vi "gds_rx_init.vi"(8 "error in (no error)":errorcluster, 10 "HW parameters In":T2={"Device IP Address"="192.168.11.6", "Active Antenna"="RX1", "Carrier Frequency (Hz)"=915000000.0, "Gain (dB)"=10.0, "Trigger Level"=0.01, "Bandwidth (Hz)"=40000000.0, "Reference Position (%)"=10.0, "Capture Time (s)"=0.0004, "Simulate"=FALSE} {"Capture Time (s)" format="%.2p"; "Bandwidth (Hz)" format="%.2p"; "Trigger Level" format="%#.3p"; "Gain (dB)" format="%.2f"; "Carrier Frequency (Hz)" format="%.2p"}, 11 "Modulation Parameters":T1) -> (0 "error out":errorcluster, 2 "HW parameters Out":T2={"Device IP Address"="192.168.11.6", "Active Antenna"="RX1", "Carrier Frequency (Hz)"=915000000.0, "Gain (dB)"=10.0, "Trigger Level"=0.01, "Bandwidth (Hz)"=40000000.0, "Reference Position (%)"=10.0, "Capture Time (s)"=0.0004, "Simulate"=FALSE} {"Capture Time (s)" format="%.2p"; "Bandwidth (Hz)" format="%.2p"; "Trigger Level" format="%#.3p"; "Gain (dB)" format="%.2f"; "Carrier Frequency (Hz)" format="%.2p"}, 3 "Modulation Parameters Out":T1)   [LabVIEW 2012]
uses:
  EE 497/LABS/SDR/control_type_defs.llb/rx_hw params.ctl
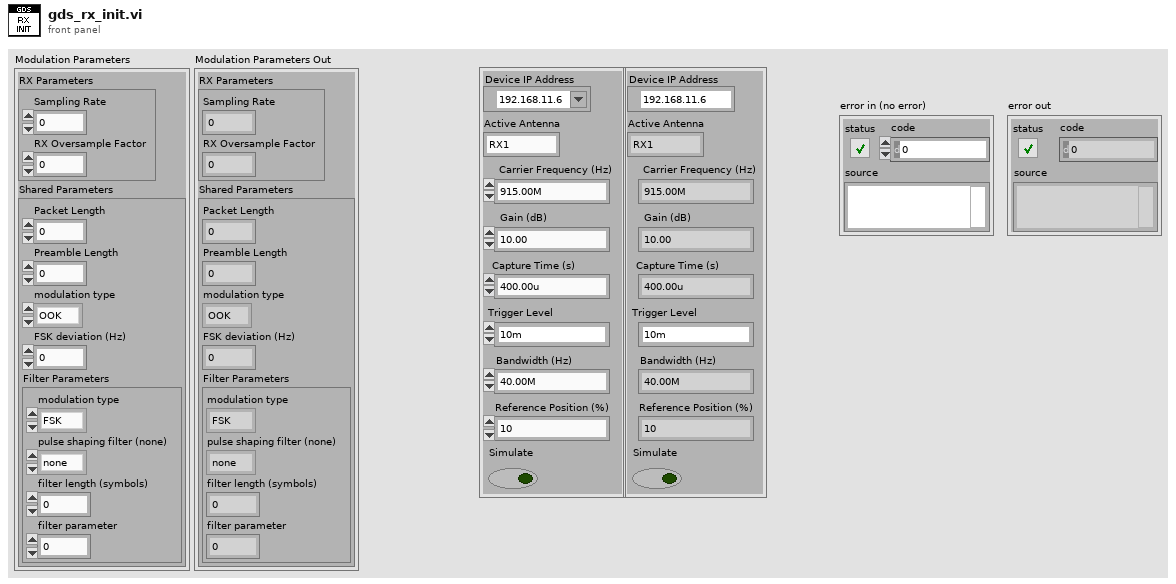
[diagram p1: front panel]
types:
  T1 = cluster{"RX Parameters":cluster{"Sampling Rate":dbl, "RX Oversample Factor":i32}, "Shared Parameters":cluster{"Packet Length":i32, "Preamble Length":i32, "modulation type":enum16{"OOK", "FSK", "PSK", "QAM", "MSK", "PAM", "ASK", "CPM"}, "FSK deviation (Hz)":dbl, "Filter Parameters":cluster{"modulation type":enum16{"FSK", "PSK", "QAM", "MSK", "PAM", "ASK", "CPM"}, "pulse shaping filter (none)":enum16{"none", "Raised Cosine", "Root Raised Cos", "Gaussian"}, "filter length (symbols)":i32, "filter parameter":dbl}}}
  T2 = typedef "rx_hw params.ctl" = cluster{"Device IP Address":refnum<k15>, "Active Antenna":string, "Carrier Frequency (Hz)":dbl, "Gain (dB)":dbl, "Trigger Level":dbl, "Bandwidth (Hz)":dbl, "Reference Position (%)":dbl, "Capture Time (s)":dbl, "Simulate":bool}
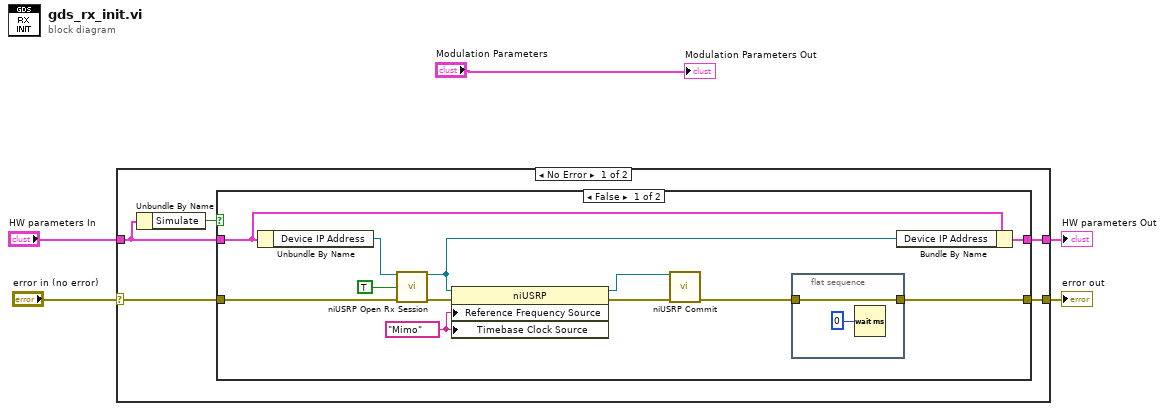
[diagram p0: block diagram]
diagram:
  n1 = case shown="No Error" "error in (no error)" {
    selector: "error in (no error)" -> [w9 w27]
    tunnel: "HW parameters In" -> [w8 w28]
    tunnel: [w7 w28] -> w3
    tunnel: [w6 w27] -> w2
    frame No Error {
      n2 = Unbundle By Name(w8) -> ("Simulate"=w10:bool)
      n3 = case shown="False" w10 {
        tunnel: w9 -> [w19 w25]
        tunnel: w8 -> [w20 w26]
        tunnel: [w18 w26] -> w7
        tunnel: [w11 w25] -> w6
        frame False {
          w15 = "Mimo" ("Clocking and Synchronization:Reference Frequency Source")
          n4 = Unbundle By Name(w20) -> ("Device IP Address"=w22:refnum<k15>)
          n5 = call <instrlib>:"niUSRP Open Rx Session.vi"("device names"=w22, "reset"=TRUE, "error in (no error)"=w19) -> ("session handle out"=w16:refnum<k15>, "error out"=w17:errorcluster)  [unwired: 11 in]
          n6 = property class="niUSRP"(reference=w16, error in=w17, "Reference Frequency Source"=w15, "Timebase Clock Source"=w15) -> (reference out=w14:refnum<k15>, error out=w13:errorcluster)
          n7 = call <instrlib>:"niUSRP Commit.vi"("session handle"=w14, "error in (no error)"=w13) -> ("error out"=w12:errorcluster)  [unwired: 12 in, 1 out]
          n8 = flat-sequence {
            tunnel: [w23] -> w11
            tunnel: w12 -> [w23]
            frame #0 {
              n9 = Wait (ms)(milliseconds to wait=u32 0) -> ()  [unwired: 1 out]
            }
          }
          n10 = Bundle By Name(cluster=w20, "Device IP Address"=w16) -> (w18:T2)
        }
        frame True {
        }
      }
    }
    frame Error {
    }
  }
  "error out" <- w2
  "HW parameters Out" <- w3
  "Modulation Parameters Out" <- "Modulation Parameters"
